vi "ifr2025 Modulation Modes  .vi"(8 "error in (no error)":errorcluster {"code" format="%.0x"}, 11 "instrument handle":refnum<visa-resource-name>) -> (0 "error out":errorcluster {"code" format="%.0x"}, 1 "Pulse":i16, 2 "Modulation Mode":i16, 3 "instrument handle out":refnum<visa-resource-name>, 4 "Global Modulation":i16, 5 "Global Pulse":i16)   [LabVIEW 2009]
doc: "Returns information about the modulation and global modes of the instrument."
uses:
  Ifr2025_32.dll
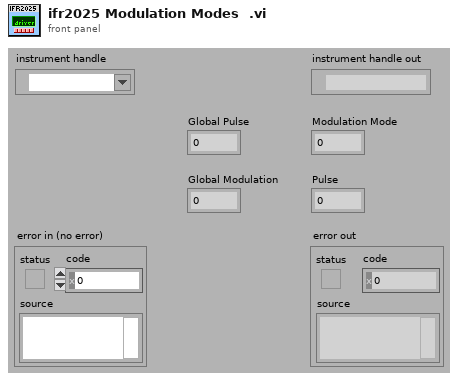
[diagram p1: front panel]
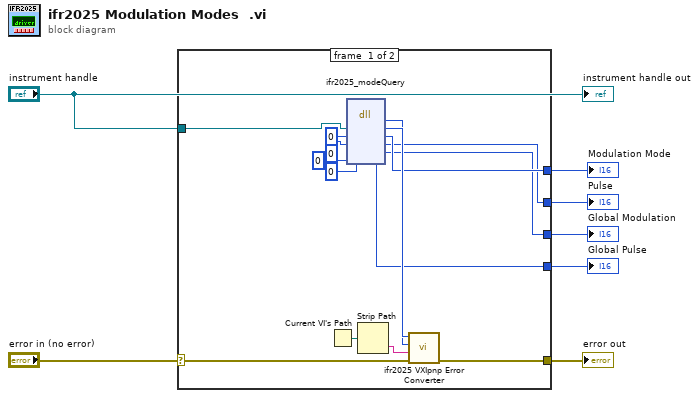
[diagram p0: block diagram]
diagram:
  n1 = case shown="No Error" "error in (no error)" {
    selector: "error in (no error)" -> [w17 w23]
    tunnel: [w16 w23] -> w7
    tunnel: "instrument handle" -> [w21 _]
    tunnel: [w14 _] -> w4
    tunnel: [w12 _] -> w3
    tunnel: [w10 _] -> w2
    tunnel: [w8 _] -> w1
    frame #0 {
      n2 = Current VI's Path() -> (path=w22:path)
      n3 = dll-call lib="P:/inst/Marconi 2024 Signal Generator/source/labview/ifr2025/ifr2025/ifr2025_*.*" fn="ifr2025_modeQuery"("vi"=w21, "Modulation Mode"=i16 0, "Pulse"=i16 0, "Global Modulation"=i16 0, "Global Pulse"=i16 0) -> (w19:i32, "vi"=w20:u32, "Modulation Mode"=w14:i16, "Pulse"=w12:i16, "Global Modulation"=w10:i16, "Global Pulse"=w8:i16)  [unwired: 3 in, 2 out]
      n4 = Strip Path(path=w22) -> (name=w18:string)  [unwired: 1 out]
      n5 = call "ifr2025 VXIpnp Error Converter.vi"("error in (no error)"=w17, "name of VI (\"\")"=w18, "CVI error code (0)"=w19, "instrument handle"=w20) -> ("error out"=w16:errorcluster)  [unwired: 7 out]
    }
    frame #1 {
    }
  }
  "error out" <- w7
  "Modulation Mode" <- w4
  "Pulse" <- w3
  "Global Modulation" <- w2
  "Global Pulse" <- w1
  "instrument handle out" <- "instrument handle"
